vi "Get_data.vi"(3 "error in (no error)":errorcluster, 4 "Input File":path) -> (0 "error out":errorcluster, 1 "Output Waveform":waveform(dbl))   [LabVIEW 2014, in "Melody Extraction.lvlib"]
uses:
  Melody Extraction.lvlib
  <vilib>/Platform/storage/lvStorage.llb/_openFunction.ctl
  <vilib>/Platform/storage/lvStorage.llb/_openStorageWithRootAutoDetect.vi
  <vilib>/Platform/storage/lvStorage.llb/xStorage/xStorageSupp/ErrorOut.vi
  <vilib>/Platform/storage/lvStorage.llb/_queryPropPoly.vi
  <vilib>/Platform/storage/lvStorage.llb/_queryPropString.vi
  <vilib>/Platform/storage/lvStorage.llb/_queryGenericObjects.vi
  <vilib>/Platform/storage/lvStorage.llb/_loadAllWaveform.vi
  <vilib>/Platform/storage/Storage.llb/Get Object Info.vi
  <vilib>/Platform/storage/Storage.llb/__closeStorageFromObject.vi
  <vilib>/Platform/storage/lvStorage.llb/xStorage/Open Data Storage/Open Data Storage.xnode
  <vilib>/Platform/storage/lvStorage.llb/xStorage/Read Data/Read Data.xnode
  <vilib>/Platform/storage/lvStorage.llb/xStorage/Close Data Storage/Close Data Storage.xnode
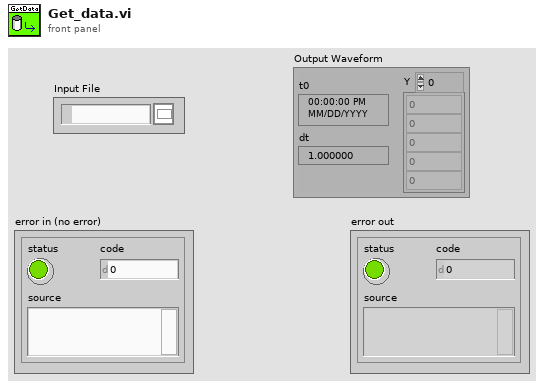
[diagram p1: front panel]
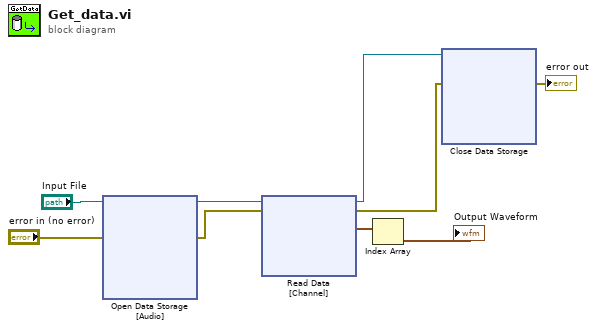
[diagram p0: block diagram]
diagram:
  n1 = xnode "Open Data Storage\n[Audio]"("file path"="Input File", "error in (no error)"="error in (no error)") -> ("storage refnum (file)"=w5:refnum<k20>, "error out"=w8:errorcluster)  [unwired: 3 in, 1 out]
  n2 = xnode "Read Data\n[Channel]"("storage refnum (file)"=w5, "error in"=w8) -> ("storage refnum (file) out"=w6:refnum<k20>, "error out"=w7:errorcluster, "Signal"=w9:waveform(dbl)[])  [unwired: 2 in, 1 out]
  n3 = Index Array(array=w9) -> (element=→"Output Waveform":waveform(dbl))  [unwired: 1 in]
  n4 = xnode "Close Data Storage\n"("storage refnum (file)"=w6, "error in (no error)"=w7) -> ("error out"=→"error out":errorcluster)  [unwired: 1 out]
